vi "Cchess.vi"() -> ()   [LabVIEW 2009]
uses:
  <vilib>/Utility/file.llb/Read From Spreadsheet File (DBL).vi
  <vilib>/Utility/file.llb/Write To Spreadsheet File (I64).vi
panel:
  out "Exit":bool
  in  "Play&Pause":bool
  in  "Next":bool
  in  "Previous":bool
  in  "Continue":bool
  in  "Review":bool
  in  "New":bool
  in  "Back":bool
  in  "Lost":bool
  in  "Initial":picture
  out "path":path
  out "Num":i32
  out "Output Array":i32[][][](array[numeric])=[[[240, 230, 220, 210, 200, 211, 221, 231, 241], [-1, -1, -1, -1, -1, -1, -1, -1, -1], [-1, 250, -1, -1, -1, -1, -1, 251, -1], [260, -1, 261, -1, 262, -1, 263, -1, 264], [-1, -1, -1, -1, -1, -1, -1, -1, -1], [-1, -1, -1, -1, -1, -1, -1, -1, -1], [160, -1, 161, -1, 162, -1, 163, -1, 164], [-1, 150, -1, -1, -1, -1, -1, 151, -1], [-1, -1, -1, -1, -1, -1, -1, -1, -1], [140, 130, 120, 110, 100, 111, 121, 131, 141]]]
  in  "Blank":picture
  out "Color":i32=1
  out "Chess":picture
  out "Board":picture
  out "Chess Array":i32[][](array[numeric])=[[240, 230, 220, 210, 200, 211, 221, 231, 241], [-1, -1, -1, -1, -1, -1, -1, -1, -1], [-1, 250, -1, -1, -1, -1, -1, 251, -1], [260, -1, 261, -1, 262, -1, 263, -1, 264], [-1, -1, -1, -1, -1, -1, -1, -1, -1], [-1, -1, -1, -1, -1, -1, -1, -1, -1], [160, -1, 161, -1, 162, -1, 163, -1, 164], [-1, 150, -1, -1, -1, -1, -1, 151, -1], [-1, -1, -1, -1, -1, -1, -1, -1, -1], [140, 130, 120, 110, 100, 111, 121, 131, 141]]
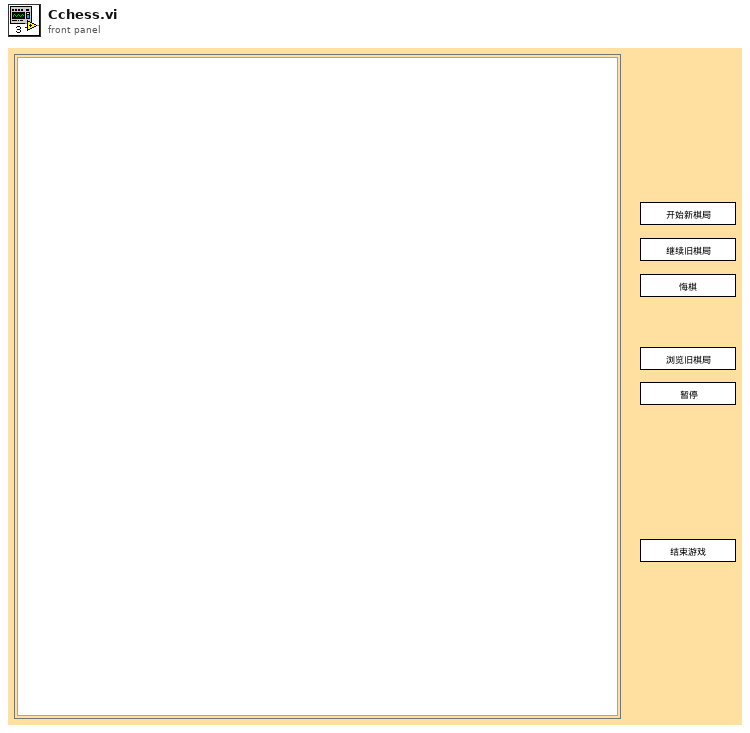
[diagram p1: front panel]
types:
  T1 = typedef "LVMouseTypeDef.ctl" = cluster{"Mouse Position":cluster{"X":i32, "Y":i32}, "Mouse Modifiers":cluster{"Button Down":bool, "Shift Mod":bool, "Menu Mod":bool, "Option Mod":bool}}
  T2 = cluster{"Left":i32, "Top":i32, "Right":i32, "Bottom":i32}
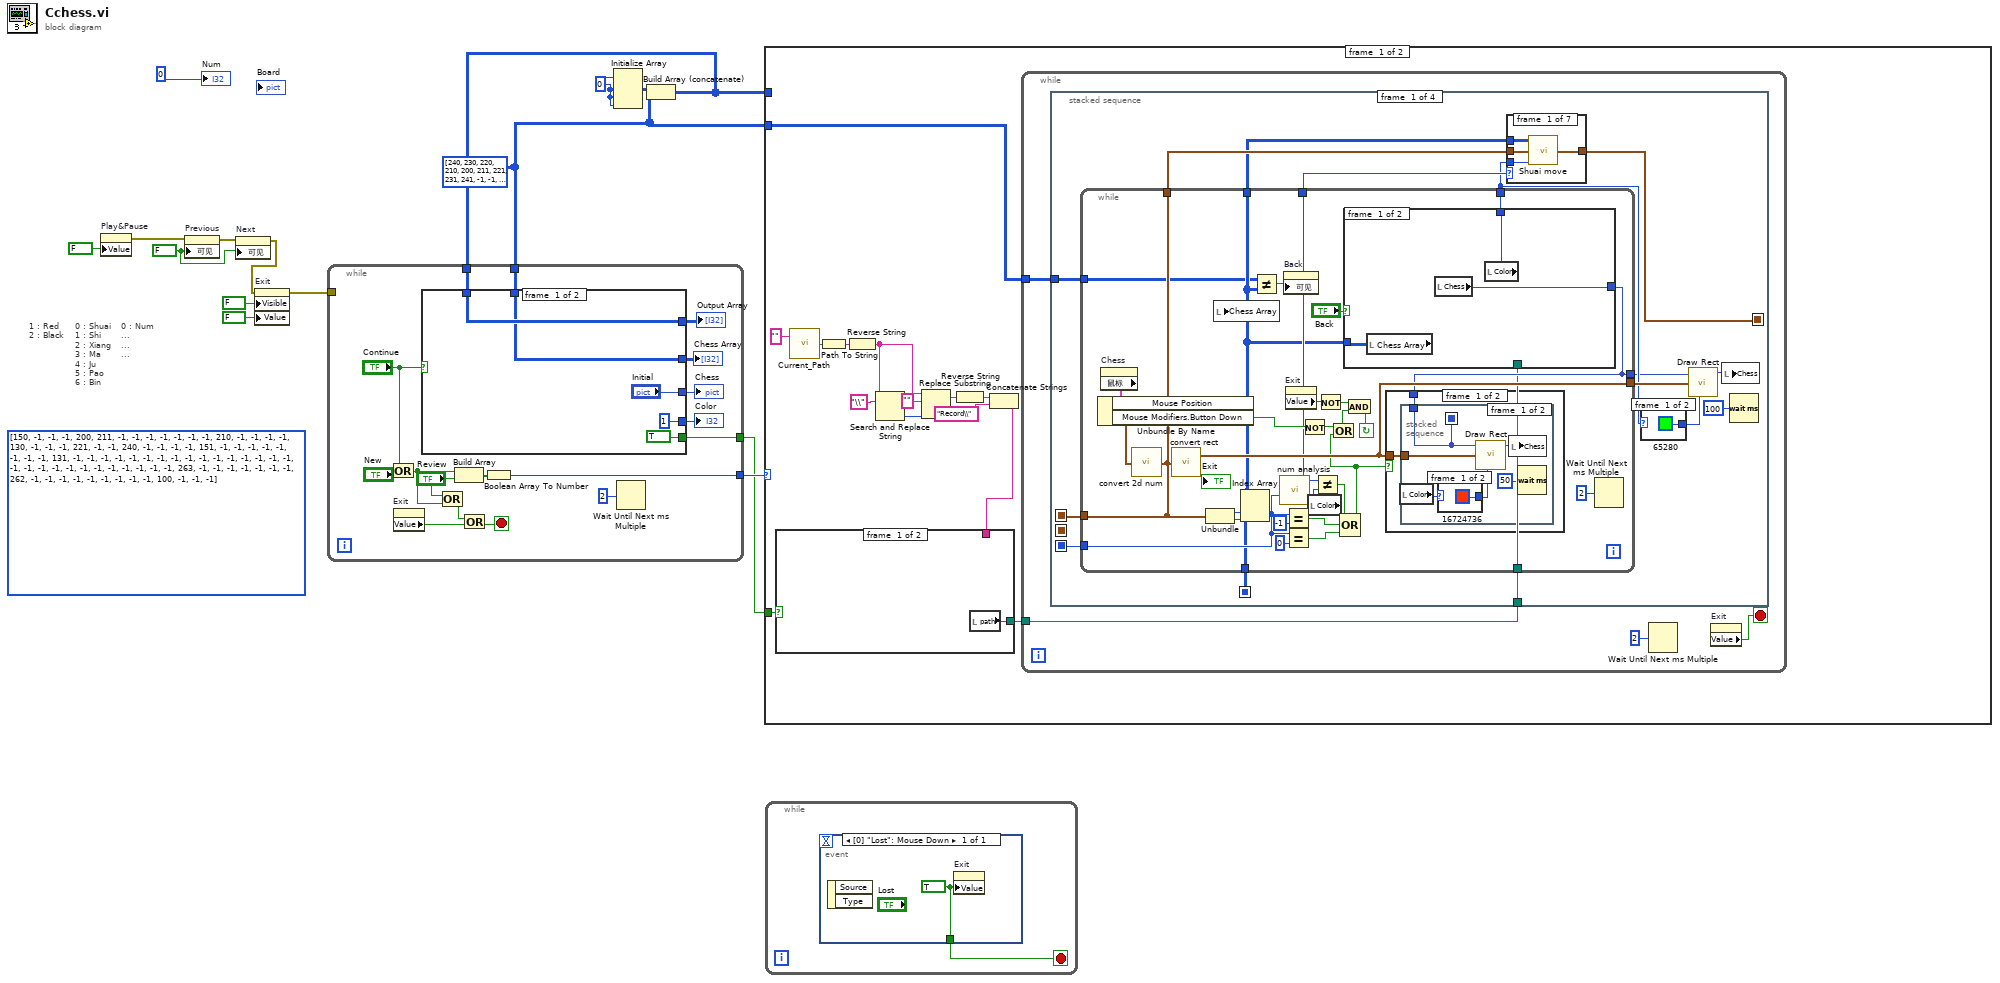
[diagram p0: block diagram]
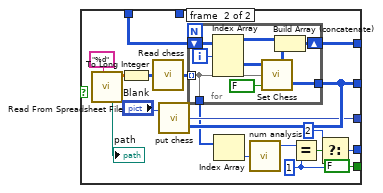
[diagram p2: hidden frame]
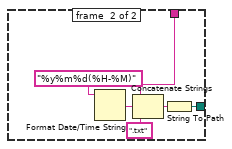
[diagram p3: hidden frame]
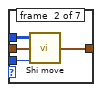
[diagram p4: hidden frame]
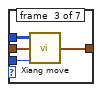
[diagram p5: hidden frame]
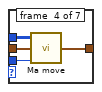
[diagram p6: hidden frame]
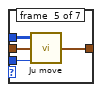
[diagram p7: hidden frame]
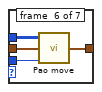
[diagram p8: hidden frame]
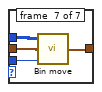
[diagram p9: hidden frame]
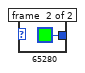
[diagram p10: hidden frame]
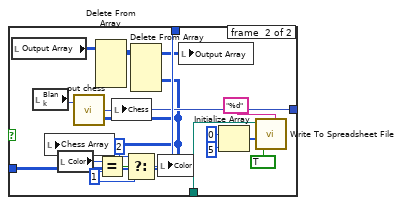
[diagram p11: hidden frame]
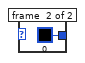
[diagram p12: hidden frame]
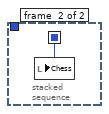
[diagram p13: hidden frame]
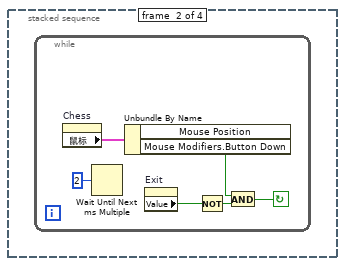
[diagram p15: hidden frame]
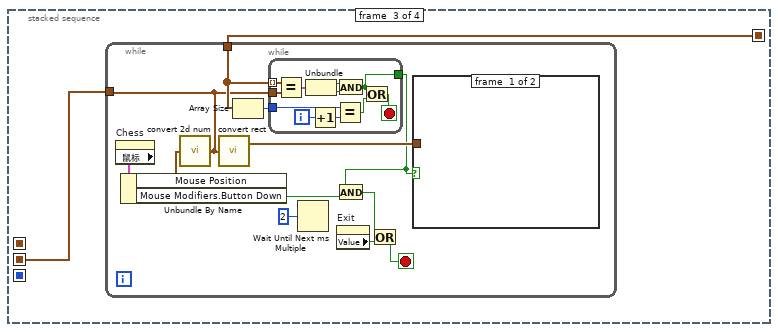
[diagram p16: hidden frame]
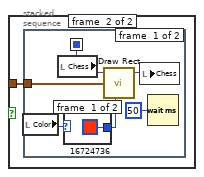
[diagram p17: hidden frame]
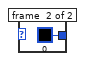
[diagram p18: hidden frame]
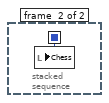
[diagram p19: hidden frame]
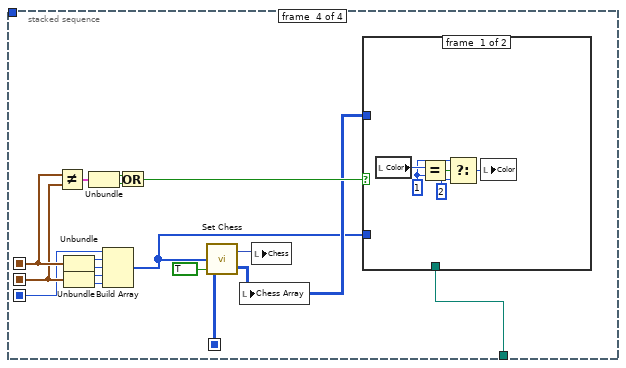
[diagram p20: hidden frame]
diagram:
  w4 = FALSE ("Visible")
  (unwired) i32[][] [[150, -1, -1, -1, 200, 211, -1, -1, -1], [-1, -1, -1, -1, 210, -1, -1, -1, -1], [130, -1, -1, -1, 221, -1, -1, 240, -1], [-1, -1, -1, 151, -1, -1, -1, -1, -1], [-1, -1, -1, 131, -1, -1, -1, -1, -1], [-1, -1, -1, -1, -1, -1, -1, -1, -1], [-1, -1, -1, -1, -1, -1, -1, -1, -1], [-1, -1, -1, -1, -1, 263, -1, -1, -1], [-1, -1, -1, -1, 262, -1, -1, -1, -1], [-1, -1, -1, -1, -1, 100, -1, -1, -1]] ("Chess Array 2")
  w9 = i32[][] [[240, 230, 220, 210, 200, 211, 221, 231, 241], [-1, -1, -1, -1, -1, -1, -1, -1, -1], [-1, 250, -1, -1, -1, -1, -1, 251, -1], [260, -1, 261, -1, 262, -1, 263, -1, 264], [-1, -1, -1, -1, -1, -1, -1, -1, -1], [-1, -1, -1, -1, -1, -1, -1, -1, -1], [160, -1, 161, -1, 162, -1, 163, -1, 164], [-1, 150, -1, -1, -1, -1, -1, 151, -1], [-1, -1, -1, -1, -1, -1, -1, -1, -1], [140, 130, 120, 110, 100, 111, 121, 131, 141]] ("Chess Array 2")
  w12 = 0 ("Dimension Size")
  # "0 : Num\n...\n...\n..."
  # "0 : Shuai\n1 : Shi\n2 : Xiang\n3 : Ma\n4 : Ju\n5 : Pao\n6 : Bin"
  # "1 : Red\n2 : Black"
  n1 = property on="Play&Pause" class="Bool (strict)"("Value"=FALSE ("Play&Pause")) -> (error out=w1:errorcluster)  [unwired: 2 in, 1 out]
  n2 = property on="Previous" class="Bool (strict)"(error in=w1, "可见"=w4) -> (error out=w5:errorcluster)  [unwired: 1 in, 1 out]
  n3 = property on="Next" class="Bool (strict)"(error in=w5, "可见"=w4) -> (error out=w3:errorcluster)  [unwired: 1 in, 1 out]
  n4 = property on="Exit" class="Bool (strict)"(error in=w3, "Visible"=FALSE, "Value"=FALSE ("Exit")) -> (error out=w8:errorcluster)  [unwired: 1 in, 1 out]
  n5 = Initialize Array(w12, w12, w12, w12) -> (w13:i32[][][])
  n6 = Build Array (concatenate)(w13, w9) -> (w14:i32[][][])
  n7 = while {
    tunnel: [w31] -> w15
    tunnel: w14 -> [w26]
    tunnel: w9 -> [w21]
    tunnel: [w20] -> w10
    tunnel: w8 -> [_]
    stop <- w16 stop-if-true
    n8 = Or(x="Continue", y="New") -> (x .or. y?=w27:bool)
    n9 = property on="Exit" class="Bool (strict)"() -> ("Value"=w17:bool)  [unwired: 2 in, 2 out]
    n10 = case shown="True" "Continue" {
      tunnel: w26 -> [w37 w51]
      tunnel: ["Initial" w48] -> w25
      tunnel: [w36 w49] -> w24
      tunnel: [w37 w47] -> w23
      tunnel: [1 ("Color") w40] -> w22
      tunnel: w21 -> [w36 _]
      tunnel: [TRUE FALSE] -> w20
      frame #0 {
      }
      frame #1 {
        w41 = 1 ("y")
        n11 = call-poly <vilib>:"Read From Spreadsheet File.vi"("format (%.3f)"="%d") -> ("all rows"=w54:dbl[][], "new file path (Not A Path if cancelled)"=→"path":path)  [unwired: 3 in, 6 out]
        n12 = To Long Integer(number=w54) -> (32bit integer=w53:i32[][])
        n13 = call "Read chess.vi"("Array"=w53) -> ("Array 2"=w52:i32[][])
        n14 = for {
          tunnel: w52 -> [w57] mode=indexing
          shift-right: [w59] -> w47
          shift-left: w51 -> [w61]
          tunnel: [w58] -> w49
          tunnel: [w57] -> w46
          i -> [w60]
          n15 = Index Array(array=w61, index (dim 0)=w60) -> (element=w56:i32[][])  [unwired: 2 in]
          n16 = call "Set Chess.vi"("Pic out"=FALSE, "Move Array"=w57, "Chess Array"=w56) -> ("Chess Array Output"=w58:i32[][])  [unwired: 1 out]
          n17 = Build Array (concatenate)(w61, w58) -> (w59:i32[][][])
        }
        n18 = call "put chess.vi"("Chess Array"=w49, "In Pic"="Blank") -> ("Out Pic"=w48:picture)
        n19 = Index Array(array=w46) -> (element=w45:i32)  [unwired: 1 in]
        n20 = call "num analysis.vi"("x"=w45) -> ("Color"=w44:i32)  [unwired: 2 out]
        n21 = Equal?(x=w44, y=w41) -> (x = y?=w43:bool)
        n22 = Select(t=2, s=w43, f=w41) -> (s? t:f=w40:i32)
      }
    }
    "Chess" <- w25
    "Chess Array" <- w24
    "Output Array" <- w23
    "Color" <- w22
    n23 = Or(x="Review", y=w27) -> (x .or. y?=w18:bool)
    n24 = Build Array(w27, "Review") -> (w32:bool[])
    n25 = Or(x=w18, y=w17) -> (x .or. y?=w16:bool)
    n26 = Boolean Array To Number(Boolean array=w32) -> (number=w31:u32)
    n27 = Wait Until Next ms Multiple(millisecond multiple=u32 2) -> ()  [unwired: 1 out]
  }
  n28 = case shown="2" w15 {
    tunnel: w9 -> [w76 _]
    tunnel: w14 -> [_ w268]
    tunnel: w10 -> [w74 _]
    frame #0 {
      n29 = call "Current_Path.vi"("Dir Or File Name"="") -> ("Dir or File In Current Path"=w72:path)  [unwired: 1 in]
      n30 = Path To String(path=w72) -> (string=w70:string)
      n31 = Reverse String(1:w70) -> (0:w68:string)
      n32 = Search and Replace String(input string=w68, search string="\\") -> (offset past replacement=w66:i32)  [unwired: 1 in, 8 out]
      n33 = Replace Substring(2:w66, 4:"" ("substring (\"\")"), 5:w68) -> (1:w65:string)  [unwired: 2 out]
      n34 = Reverse String(1:w65) -> (0:w64:string)
      n35 = Concatenate Strings(w64, "Record\\" ("Substring")) -> (w63:string)
      n36 = case shown="True" w74 {
        tunnel: [w77 w79] -> w75
        tunnel: w63 -> [_ w78]
        frame #0 {
          n37 = local read "path"() -> (w77:path)
        }
        frame #1 {
          n38 = Format Date/Time String(time format string (%c)="%y%m%d(%H-%M)") -> (date/time string=w83:string)  [unwired: 2 out]
          n39 = Concatenate Strings(w78, w83, ".txt") -> (w81:string)
          n40 = String To Path(string=w81) -> (path=w79:path)
        }
      }
      n41 = while {
        tunnel: w75 -> [w87]
        tunnel: w76 -> [w86]
        stop <- w84 stop-if-true
        n42 = stacked-sequence {
          seq-local: [w102 _ _ _] -> [_ _ _ w246]
          seq-local: [w101 _ _ _] -> [_ _ _ w244]
          seq-local: [w95 _ _ _] -> [_ _ w200 _]
          seq-local: [_ _ w199 _] -> [_ _ _ w245]
          seq-local: [w93 _ _ _] -> [_ _ _ w238]
          tunnel: w87 -> [w89 _ _ w235]
          tunnel: w86 -> [w88 _ _ _]
          frame #0 {
            n43 = while {
              tunnel: [w157] -> w97
              tunnel: [w151] -> w102
              tunnel: [w149] -> w101
              tunnel: [w151] -> w94
              tunnel: [w146] -> w96
              tunnel: [w141] -> w93
              tunnel: [w141] -> w90
              tunnel: [w143] -> w92
              tunnel: [w142] -> w91
              tunnel: w89 -> [w139]
              tunnel: w88 -> [w138]
              stop <- w133 continue-if-true
              n44 = property on="Chess" class="Picture"() -> ("鼠标"=w158:T1)  [unwired: 2 in, 2 out]
              n45 = Unbundle By Name(w158) -> ("Mouse Position"=w162:cluster{"X":i32, "Y":i32}, "Mouse Modifiers.Button Down"=w154:bool)
              n46 = call "convert 2d num.vi"("Mouse Position"=w162) -> ("Array Position"=w151:cluster{"Row":i32, "Column":i32})
              n47 = call "convert rect.vi"("Array Position"=w151) -> ("Output Rect"=w157:T2)  [unwired: 1 out]
              n48 = Unbundle(w151) -> ("Row"=w161:i32, "Column"=w160:i32)
              n49 = property on="Exit" class="Bool (strict)"() -> ("Value"=w135:bool)  [unwired: 2 in, 2 out]
              n50 = Not(x=w154) -> (.not. x?=w153:bool)
              n51 = local read "Color"() -> (w156:i32)
              n52 = Not(x=w135) -> (.not. x?=w136:bool)
              n53 = case shown="True" "Back" {
                tunnel: [w164 w166] -> w141
                tunnel: [w165 w177] -> w143
                tunnel: [w163 w175] -> w142
                tunnel: w139 -> [_ w169]
                frame #0 {
                  n54 = local read "Chess Array"() -> (w164:i32[][])
                  n55 = local read "Chess"() -> (w163:picture)
                  n56 = local read "Color"() -> (w165:i32)
                }
                frame #1 {
                  w179 = 1 ("y")
                  n57 = local read "Output Array"() -> (w168:i32[][][])
                  n58 = local read "Blank"() -> (w181:picture)
                  n59 = local read "Color"() -> (w180:i32)
                  n60 = Delete From Array(array=w168) -> (array with subset deleted=w167:i32[][][])  [unwired: 4 in, 1 out]
                  n61 = Equal?(x=w180, y=w179) -> (x = y?=w178:bool)
                  n62 = Select(t=2, s=w178, f=w179) -> (s? t:f=w177:i32)
                  n63 = Delete From Array(array=w167) -> (deleted portion=w166:i32[][])  [unwired: 4 in, 1 out]
                  n64 = local write "Chess Array"(w166) -> ()
                  n65 = call "put chess.vi"("Chess Array"=w166, "In Pic"=w181) -> ("Out Pic"=w175:picture)
                  n66 = local write "Chess"(w175) -> ()
                  n67 = local write "Color"(w177) -> ()
                  n68 = local write "Output Array"(w167) -> ()
                  n69 = Initialize Array(0 ("Element Data"), 5 ("Dimension Size")) -> (w170:i32[])
                  n70 = call-poly <vilib>:"Write To Spreadsheet File.vi"("format (%d)"="%d" ("format (%.3f)"), "append to file? (new file:F)"=TRUE, "1D data"=w170, "file path (dialog if empty)"=w169) -> ()  [unwired: 2 in, 3 out]
                }
              }
              n71 = local write "Chess Array"(w141) -> ()
              n72 = Index Array(array=w141, index (row)=w161, index (col)=w160) -> (element=w149:i32)
              n73 = Not Equal?(x=w138, y=w141) -> (x != y?=w140:bool)
              n74 = call "num analysis.vi"("x"=w149) -> ("Color"=w145:i32, "Chess"=w146:i32)  [unwired: 1 out]
              n75 = property on="Back" class="Boolean (strict)"("可见"=w140) -> ()  [unwired: 2 in, 2 out]
              n76 = Equal?(x=w149, y=-1) -> (x = y?=w150:bool)
              n77 = Equal?(x=w149, y=0) -> (x = y?=w147:bool)
              n78 = Not Equal?(x=w145, y=w156) -> (x != y?=w155:bool)
              n79 = Compound Arithmetic op=OR(w155, w150, w147) -> (w152:bool)
              n80 = Or(x=w153, y=w152) -> (x .or. y?=w134:bool)
              n81 = And(x=w136, y=w134) -> (x .and. y?=w133:bool)
              n82 = case shown="True" w152 {
                tunnel: w157 -> [w183 _]
                tunnel: w142 -> [w182 _]
                frame #0 {
                  n83 = stacked-sequence {
                    seq-local: [w184 _] -> [_ w192]
                    tunnel: w183 -> [w186 _]
                    tunnel: w182 -> [w184 _]
                    frame #0 {
                      n84 = local read "Color"() -> (w185:i32)
                      n85 = case shown="1, Default" w185 {
                        tunnel: [u32 16724736 ("color(black)") u32 0 ("color(black)")] -> w189
                        frame #0 {
                        }
                        frame #1 {
                        }
                      }
                      n86 = call <vilib>:"Draw Rect.vi"("picture"=w184, "rect"=w186, "color(black)"=w189) -> ("new picture"=w188:picture)  [unwired: 4 in, 2 out]
                      n87 = local write "Chess"(w188) -> ()
                      n88 = Wait (ms)(milliseconds to wait=u32 50) -> ()  [unwired: 1 out]
                    }
                    frame #1 {
                      n89 = local write "Chess"(w192) -> ()
                    }
                  }
                }
                frame #1 {
                }
              }
              n90 = Wait Until Next ms Multiple(millisecond multiple=u32 2) -> ()  [unwired: 1 out]
            }
            n91 = case shown="1" w96 {
              tunnel: [w103 w107 w111 w115 w121 w124 w127] -> w95
              tunnel: w90 -> [w106 w110 w114 w118 w120 w126 w130]
              tunnel: w92 -> [w104 w108 w113 w117 w119 w125 w128]
              tunnel: w94 -> [w105 w109 w112 w116 w122 w123 w129]
              frame #0 {
                n92 = call "Shuai move.vi"("Color"=w104, "Array Position"=w105, "Chess Array"=w106) -> ("Shuai move"=w103:cluster{i32, i32}[])
              }
              frame #1 {
                n93 = call "Shi move.vi"("Color"=w108, "Array Position"=w109, "Chess Array"=w110) -> ("Shi move"=w107:cluster{i32, i32}[])
              }
              frame #2 {
                n94 = call "Xiang move.vi"("Color"=w113, "Array Position"=w112, "Chess Array"=w114) -> ("Xiang move"=w111:cluster{i32, i32}[])
              }
              frame #3 {
                n95 = call "Ma move.vi"("Color"=w117, "Array Position"=w116, "Chess Array"=w118) -> ("Ma move"=w115:cluster{i32, i32}[])
              }
              frame #4 {
                n96 = call "Ju move.vi"("Color"=w119, "Array Position"=w122, "Chess Array"=w120) -> ("Ju move"=w121:cluster{"Row":i32, i32}[])
              }
              frame #5 {
                n97 = call "Pao move.vi"("Color"=w125, "Array Position"=w123, "Chess Array"=w126) -> ("Ju move"=w124:cluster{"Row":i32, i32}[])
              }
              frame #6 {
                n98 = call "Bin move.vi"("Color"=w128, "Array Position"=w129, "Chess Array"=w130) -> ("Shuai move"=w127:cluster{i32, i32}[])
              }
            }
            n99 = case shown="1, Default" w92 {
              tunnel: [u32 65280 ("color(black)") u32 65280 ("color(black)")] -> w98
              frame #0 {
              }
              frame #1 {
              }
            }
            n100 = call <vilib>:"Draw Rect.vi"("picture"=w91, "rect"=w97, "color(black)"=w98) -> ("new picture"=w99:picture)  [unwired: 4 in, 2 out]
            n101 = local write "Chess"(w99) -> ()
            n102 = Wait (ms)(milliseconds to wait=u32 100) -> ()  [unwired: 1 out]
          }
          frame #1 {
            n103 = while {
              stop <- w193 continue-if-true
              n104 = property on="Chess" class="Picture"() -> ("鼠标"=w198:T1)  [unwired: 2 in, 2 out]
              n105 = Wait Until Next ms Multiple(millisecond multiple=u32 2) -> ()  [unwired: 1 out]
              n106 = Unbundle By Name(w198) -> ("Mouse Modifiers.Button Down"=w194:bool)  [unwired: 1 out]
              n107 = property on="Exit" class="Bool (strict)"() -> ("Value"=w196:bool)  [unwired: 2 in, 2 out]
              n108 = Not(x=w196) -> (.not. x?=w195:bool)
              n109 = And(x=w194, y=w195) -> (x .and. y?=w193:bool)
            }
          }
          frame #2 {
            n110 = while {
              tunnel: w200 -> [w209]
              tunnel: [w207] -> w199
              stop <- w201 stop-if-true
              n111 = property on="Chess" class="Picture"() -> ("鼠标"=w210:T1)  [unwired: 2 in, 2 out]
              n112 = Unbundle By Name(w210) -> ("Mouse Position"=w211:cluster{"X":i32, "Y":i32}, "Mouse Modifiers.Button Down"=w206:bool)
              n113 = call "convert 2d num.vi"("Mouse Position"=w211) -> ("Array Position"=w207:cluster{"Row":i32, "Column":i32})
              n114 = call "convert rect.vi"("Array Position"=w207) -> ("Output Rect"=w212:T2)  [unwired: 1 out]
              n115 = Array Size(array=w209) -> (size(s)=w208:i32)
              n116 = while {
                tunnel: w209 -> [w214] mode=indexing
                tunnel: w207 -> [w213]
                tunnel: [w215] -> w205
                tunnel: w208 -> [w219]
                i -> [w220]
                stop <- w217 stop-if-true
                n117 = Equal?(x=w214, y=w213) -> (x = y?=w221:cluster{"Row":bool, bool})
                n118 = Unbundle(w221) -> ("Row"=w222:bool, w223:bool)
                n119 = Increment(x=w220) -> (x+1=w218:i32)
                n120 = Equal?(x=w219, y=w218) -> (x = y?=w216:bool)
                n121 = And(x=w222, y=w223) -> (x .and. y?=w215:bool)
                n122 = Or(x=w215, y=w216) -> (x .or. y?=w217:bool)
              }
              n123 = Wait Until Next ms Multiple(millisecond multiple=u32 2) -> ()  [unwired: 1 out]
              n124 = And(x=w205, y=w206) -> (x .and. y?=w202:bool)
              n125 = property on="Exit" class="Bool (strict)"() -> ("Value"=w203:bool)  [unwired: 2 in, 2 out]
              n126 = Or(x=w202, y=w203) -> (x .or. y?=w201:bool)
              n127 = case shown="True" w205 {
                tunnel: w212 -> [_ w224]
                frame #0 {
                }
                frame #1 {
                  n128 = stacked-sequence {
                    seq-local: [w230 _] -> [_ w233]
                    tunnel: w224 -> [w226 _]
                    frame #0 {
                      n129 = local read "Color"() -> (w225:i32)
                      n130 = local read "Chess"() -> (w230:picture)
                      n131 = case shown="1, Default" w225 {
                        tunnel: [u32 16724736 ("color(black)") u32 0 ("color(black)")] -> w229
                        frame #0 {
                        }
                        frame #1 {
                        }
                      }
                      n132 = call <vilib>:"Draw Rect.vi"("picture"=w230, "rect"=w226, "color(black)"=w229) -> ("new picture"=w228:picture)  [unwired: 4 in, 2 out]
                      n133 = local write "Chess"(w228) -> ()
                      n134 = Wait (ms)(milliseconds to wait=u32 50) -> ()  [unwired: 1 out]
                    }
                    frame #1 {
                      n135 = local write "Chess"(w233) -> ()
                    }
                  }
                }
              }
            }
          }
          frame #3 {
            n136 = Not Equal?(x=w246, y=w245) -> (x != y?=w250:cluster{"Row":bool, "Column":bool})
            n137 = Unbundle(w246) -> ("Row"=w243:i32, "Column"=w242:i32)
            n138 = Unbundle(w245) -> ("Row"=w241:i32, "Column"=w240:i32)
            n139 = Unbundle(w250) -> ("Row"=w249:bool, "Column"=w248:bool)
            n140 = Build Array(w244, w243, w242, w241, w240) -> (w234:i32[])
            n141 = Or(x=w249, y=w248) -> (x .or. y?=w247:bool)
            n142 = call "Set Chess.vi"("Pic out"=TRUE, "Move Array"=w234, "Chess Array"=w238) -> ("Chess Array Output"=w237:i32[][], "Chess"=w239:picture)
            n143 = local write "Chess Array"(w237) -> ()
            n144 = local write "Chess"(w239) -> ()
            n145 = case shown="True" w247 {
              tunnel: w237 -> [_ w260]
              tunnel: w235 -> [_ w257]
              tunnel: w234 -> [_ w256]
              frame #0 {
                w251 = 1 ("y")
                n146 = local read "Color"() -> (w255:i32)
                n147 = Equal?(x=w255, y=w251) -> (x = y?=w254:bool)
                n148 = Select(t=w251, s=w254, f=2 ("t")) -> (s? t:f=w253:i32)
                n149 = local write "Color"(w253) -> ()
              }
              frame #1 {
                w266 = 1 ("y")
                n150 = local read "Output Array"() -> (w261:i32[][][])
                n151 = local read "Color"() -> (w267:i32)
                n152 = Equal?(x=w267, y=w266) -> (x = y?=w265:bool)
                n153 = Select(t=2, s=w265, f=w266) -> (s? t:f=w263:i32)
                n154 = Build Array (concatenate)(w261, w260) -> (w262:i32[][][])
                n155 = local write "Color"(w263) -> ()
                n156 = call-poly <vilib>:"Write To Spreadsheet File.vi"("format (%d)"="%d" ("format (%.3f)"), "append to file? (new file:F)"=TRUE, "1D data"=w256, "file path (dialog if empty)"=w257) -> ()  [unwired: 2 in, 3 out]
                n157 = local write "Output Array"(w262) -> ()
              }
            }
          }
        }
        n158 = Wait Until Next ms Multiple(millisecond multiple=u32 2) -> ()  [unwired: 1 out]
        n159 = property on="Exit" class="Bool (strict)"() -> ("Value"=w84:bool)  [unwired: 2 in, 2 out]
      }
    }
    frame #1 {
      n160 = call-poly <vilib>:"Read From Spreadsheet File.vi"("format (%.3f)"="%d") -> ("all rows"=w273:dbl[][])  [unwired: 3 in, 7 out]
      n161 = To Long Integer(number=w273) -> (32bit integer=w270:i32[][])
      n162 = call "Read chess.vi"("Array"=w270) -> ("Array 2"=w269:i32[][])
      n163 = Array Size(array=w269) -> (size(s)=w272:i32[])
      n164 = Index Array(array=w272) -> (element=w271:i32)  [unwired: 1 in]
      n165 = while {
        tunnel: w269 -> [w283]
        tunnel: w271 -> [w281]
        shift-right: [w278] -> _
        shift-left: w268 -> [w279]
        i -> [w282]
        stop <- w277 stop-if-true
        n166 = stacked-sequence {
          tunnel: w283 -> [_ _ w317]
          tunnel: w279 -> [_ _ w309]
          tunnel: [_ _ w305] -> w278
          frame #0 {
            n167 = case shown="True" "Play&Pause" {
              frame #0 {
                w285 = FALSE ("Visible")
                n168 = property on="Next" class="Bool (strict)"("可见"=w285) -> ()  [unwired: 2 in, 2 out]
                n169 = property on="Previous" class="Bool (strict)"("可见"=w285) -> ()  [unwired: 2 in, 2 out]
              }
              frame #1 {
                n170 = while {
                  stop <- w298 stop-if-true
                  n171 = local read "Play&Pause"() -> (w297:bool)
                  n172 = property on="Exit" class="Bool (strict)"() -> ("Value"=w293:bool)  [unwired: 2 in, 2 out]
                  n173 = Not(x=w297) -> (.not. x?=w296:bool)
                  n174 = case shown="True" "Previous" {
                    frame #0 {
                    }
                    frame #1 {
                      n175 = local read "Num"() -> (w301:i32)
                      n176 = Subtract(x=w301, y=2) -> (x-y=w299:i32)
                      n177 = local write "Num"(w299) -> ()
                    }
                  }
                  n178 = Compound Arithmetic op=OR(w293, "Next", "Previous", w296) -> (w298:bool)
                }
                n179 = local read "Num"() -> (w290:i32)
                n180 = Greater?(x=w290, y=1) -> (0:w288:bool)
                n181 = case shown="True" w288 {
                  tunnel: [FALSE ("Visible") TRUE ("Visible")] -> w287
                  frame #0 {
                  }
                  frame #1 {
                  }
                }
                n182 = property on="Next" class="Bool (strict)"("可见"=TRUE ("Visible")) -> ()  [unwired: 2 in, 2 out]
                n183 = property on="Previous" class="Bool (strict)"("可见"=w287) -> ()  [unwired: 2 in, 2 out]
              }
            }
          }
          frame #1 {
            n184 = while {
              stop <- w302 continue-if-true
              n185 = local read "Previous"() -> (w304:bool)
              n186 = local read "Next"() -> (w303:bool)
              n187 = Or(x=w304, y=w303) -> (x .or. y?=w302:bool)
            }
          }
          frame #2 {
            n188 = local read "Num"() -> (w312:i32)
            n189 = Index Array(array=w309, index (dim 0)=w312) -> (element=w311:i32[][])  [unwired: 2 in]
            n190 = Index Array(array=w317, index (row)=w312) -> (element=w314:i32[])  [unwired: 1 in]
            n191 = Increment(x=w312) -> (x+1=w313:i32)
            n192 = call "Set Chess.vi"("Pic out"=TRUE, "Move Array"=w314, "Chess Array"=w311) -> ("Chess Array Output"=w310:i32[][], "Chess"=w318:picture)
            n193 = local write "Num"(w313) -> ()
            n194 = local write "Chess"(w318) -> ()
            n195 = Array Size(array=w309) -> (size(s)=w308:i32[])
            n196 = Index Array(array=w308) -> (element=w307:i32)  [unwired: 1 in]
            n197 = Equal?(x=w307, y=w313) -> (x = y?=w306:bool)
            n198 = case shown="True" w306 {
              tunnel: w310 -> [_ w322]
              tunnel: w309 -> [w319 w321]
              tunnel: [w319 w320] -> w305
              frame #0 {
              }
              frame #1 {
                n199 = Build Array (concatenate)(w321, w322) -> (w320:i32[][][])
              }
            }
            n200 = Wait (ms)(milliseconds to wait=u32 500) -> ()  [unwired: 1 out]
          }
        }
        n201 = Increment(x=w282) -> (x+1=w280:i32)
        n202 = Equal?(x=w281, y=w280) -> (x = y?=w276:bool)
        n203 = property on="Exit" class="Bool (strict)"() -> ("Value"=w275:bool)  [unwired: 2 in, 2 out]
        n204 = Or(x=w276, y=w275) -> (x .or. y?=w277:bool)
      }
    }
  }
  n205 = while {
    stop <- w323 stop-if-true
    n206 = event shown="[0] \"Lost\": Mouse Down" {
      selector: _ -> [_]
      dyn-events: _ -> [_]
      timeout: _ -> [_]
      tunnel: [w324] -> w323
      event [0] "Lost": Mouse Down {
        w324 = TRUE ("Exit")
        n207 = event-data() -> ()  [unwired: 3 out]
        n208 = property on="Exit" class="Bool (strict)"("Value"=w324) -> ()  [unwired: 2 in, 2 out]
      }
    }
  }
  "Num" <- 0
